vi "Centauro Temp Option Knob.vi"(0 "GEA2 Reference In":refnum<k24>, 5 "Select Heat":enum16{"High", "Medium", "Low", "No Heat"}(ring), 11 "Error In":errorcluster, 12 "Verify ERD Response?":bool=TRUE) -> (4 "GEA2 Reference Out":refnum<k24>, 15 "Error Out":errorcluster)   [LabVIEW 2016]
uses:
  Q:/Common/DLLs/GEA3/GeaCommunication.dll
  Common/DLLs/GEA3/GeaCommunication.dll
  Common/LabVIEW GEA2 Toolkit/LabVIEW_GEA2_Toolkit.lvlibp/type defs/Source_Destination.ctl
  Common/LabVIEW GEA2 Toolkit/LabVIEW_GEA2_Toolkit.lvlibp/type defs/ERD Write Data In.ctl
  Common/LabVIEW GEA2 Toolkit/LabVIEW_GEA2_Toolkit.lvlibp/type defs/Data Type.ctl
  Common/LabVIEW GEA2 Toolkit/LabVIEW_GEA2_Toolkit.lvlibp
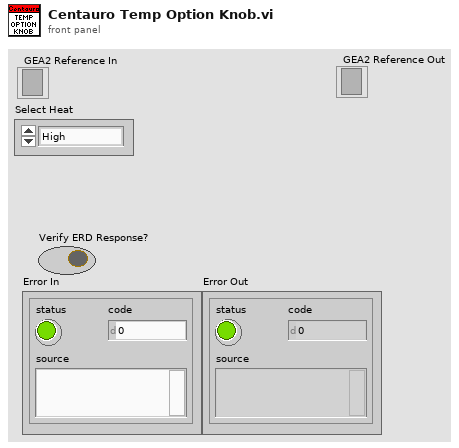
[diagram p1: front panel]
types:
  T1 = typedef "LabVIEW_GEA2_Toolkit.lvlibp/ERD Write Data In.ctl" = cluster{"ERD Number":u16, "Data Type":T2, "Data":string}
  T2 = typedef "LabVIEW_GEA2_Toolkit.lvlibp/Data Type.ctl" = enum16{"string", "boolean", "uint8_t", "uint16_t", "uint32_t", "uint64_t", "int8_t", "int16_t", "int32_t", "int64_t"}
  T3 = typedef "LabVIEW_GEA2_Toolkit.lvlibp/Source_Destination.ctl" = cluster{"Source":u8, "Destination":u8}
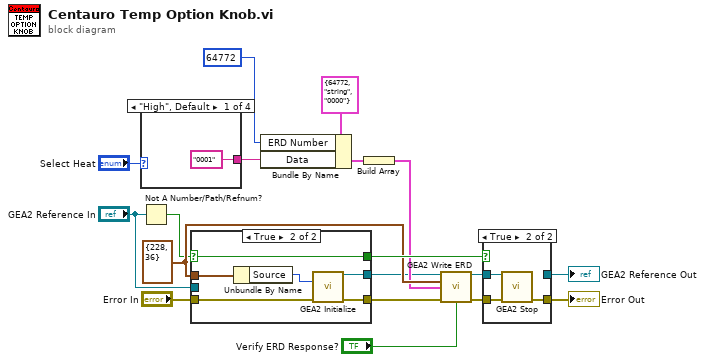
[diagram p0: block diagram]
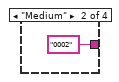
[diagram p4: hidden frame]
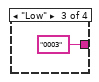
[diagram p5: hidden frame]
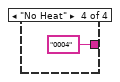
[diagram p6: hidden frame]
diagram:
  w15 = T3 {"Source"=228, "Destination"=36} ("GEA Inputs")
  n1 = case shown="\"High\", Default" "Select Heat" {
    tunnel: ["0001" "0002" "0003" "0004"] -> w7
    frame "High", Default {
    }
    frame "Medium" {
    }
    frame "Low" {
    }
    frame "No Heat" {
    }
  }
  n2 = Not A Number/Path/Refnum?(number/path/refnum="GEA2 Reference In") -> (NaN/Path/Refnum?=w14:bool)
  n3 = case shown="True" w14 {
    selector: w14 -> [w23 w26]
    tunnel: "Error In" -> [w24 w31]
    tunnel: [w24 w30] -> w8
    tunnel: "GEA2 Reference In" -> [w25 _]
    tunnel: [w25 w29] -> w4
    tunnel: w15 -> [_ w27]
    tunnel: [w23 w26] -> w16
    frame False {
    }
    frame True {
      n4 = Unbundle By Name(w27) -> ("Source"=w28:u8)
      n5 = call "GEA2 Initialize.vi"("Source Address"=w28, "error in"=w31) -> ("GEA2 Reference Out"=w29:refnum<k24>, "error out"=w30:errorcluster)  [unwired: 11 in, 1 out]
    }
  }
  n6 = Bundle By Name(cluster=T1 {"ERD Number"=64772, "Data Type"=enum."string", "Data"="0000"} ("ERD Write Data In"), "ERD Number"=u16 64772, "Data"=w7) -> (w6:T1)
  n7 = Build Array(w6) -> (w5:T1[])
  n8 = call "GEA2 Write ERD.vi"("GEA2 Reference In"=w4, "GEA Inputs"=w15, "Write ERD List"=w5, "Error In"=w8, "Verify ERD Response?"="Verify ERD Response?") -> ("GEA2 Reference Out"=w12:refnum<k24>, "Error Out"=w17:errorcluster)  [unwired: 8 in, 1 out]
  n9 = case shown="True" w16 {
    tunnel: [w32 w36] -> w10
    tunnel: w12 -> [w33 w35]
    tunnel: [w33 _] -> w11
    tunnel: w17 -> [w32 w34]
    frame False {
    }
    frame True {
      n10 = call "GEA2 Stop.vi"("GEA2 Reference In"=w35, "Error In"=w34) -> ("Error Out"=w36:errorcluster)  [unwired: 13 in]
    }
  }
  "Error Out" <- w10
  "GEA2 Reference Out" <- w11
